vi "API_Set Cursor Pos.vi"(8 "错误输入（无错误）":errorcluster, 10 "y":i32, 11 "x":i32) -> (0 "错误输出":errorcluster)   [LabVIEW 2012, in "API.lvlib"]
uses:
  API.lvlib
  user32.dll
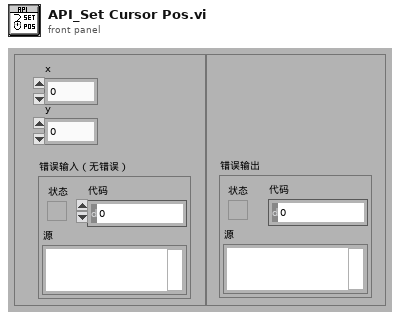
[diagram p1: front panel]
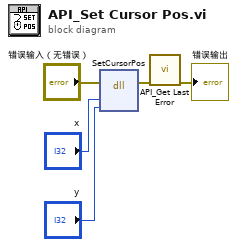
[diagram p0: block diagram]
diagram:
  n1 = dll-call lib="user32.dll" fn="SetCursorPos"(error in="错误输入（无错误）", "x"="x", "y"="y") -> (error out=w2:errorcluster)  [unwired: 5 in, 1 out]
  n2 = call "API_Get Last Error.vi"("错误输入（无错误）"=w2) -> ("错误输出"=→"错误输出":errorcluster)  [unwired: 10 in]
